vi "test_F9P_fgv-ver.vi"() -> ()   [LabVIEW 2019] (continued)
3,28,14,13,11,33,08,10,,,,,,1.19,0.67,0.98,4*09\r\n$GPGSV,4,1,13,02,65,334,42,04,08,037,40,05,48,261,36,06,58,076,45,1*6E\r\n$GPGSV,4,2,13,07,06,105,28,09,38,057,42,12,18,263,24,13,08,191,23,1*60\r\n$GPGSV,4,3,13,17,19,158,26,19,37,161,32,25,11,294,,29,07,323,19,1*62\r\n$GPGSV,4,4,13,30,01,134,,1*52\r\n$GPGSV,4,1,13,02,65,334,,04,08,037,30,05,48,261,32,06,58,076,34,6*6A\r\n$GPGSV,4,2,13,07,06,105,,09,38,057,35,12,18,263,12,13,08,191,,6*69\r\n$GPGSV,4,3,13,17,19,158,17,19,37,161,,25,11,294,,29,07,323,,6*6E\r\n$GPGSV,4,4,13,30,01,134,,6*55\r\n$GLGSV,2,1,06,70,55,030,35,71,68,223,28,72,17,216,42,84,09,133,10,1*7B\r\n$GLGSV,2,2,06,85,63,111,31,86,51,337,,1*78\r\n$GLGSV,2,1,06,70,55,030,,71,68,223,18,72,17,216,24,84,09,133,08,3*75\r\n$GLGSV,2,2,06,85,63,111,25,86,51,337,,3*7F\r\n$GAGSV,3,1,09,02,04,287,09,04,68,085,36,09,44,196,28,11,78,037,39,7*74\r\n$GAGSV,3,2,09,12,32,114,31,18,55,284,35,19,17,042,37,25,01,241,,7*73\r\n$GAGSV,3,3,09,36,35,314,23,7*4E\r\n$GAGSV,3,1,09,02,04,287,,04,68,085,35,09,44,196,26,11,78,037,33,2*7F\r\n$GAGSV,3,2,09,12,32,114,35,18,55,284,31,19,17,042,29,25,01,241,,2*79\r\n$GAGSV,3,3,09,36,35,314,26,2*4E\r\n$GBGSV,4,1,13,04,35,133,,05,09,257,,06,27,182,,07,09,201,21,1*78\r\n$GBGSV,4,2,13,08,65,355,40,09,07,194,,10,16,222,23,11,38,142,31,1*77\r\n$GBGSV,4,3,13,13,50,314,38,14,77,038,42,28,58,310,37,33,72,237,30,1*70\r\n$GBGSV,4,4,13,34,13,141,,1*45\r\n$GBGSV,4,1,13,04,35,133,,05,09,257,,06,27,182,,07,09,201,,3*79\r\n$GBGSV,4,2,13,08,65,355,39,09,07,194,,10,16,222,21,11,38,142,33,3*7B\r\n$GBGSV,4,3,13,13,50,314,39,14,77,038,36,28,58,310,,33,72,237,,3*77\r\n$GBGSV,4,4,13,34,13,141,,3*47\r\n$GNGLL,3723.61598,N,12656.96764,E,064242.00,A,A*7B\r\n$GNRMC,064243.00,A,3723.61604,N,12656.96767,E,0.173,,250720,,,A,V*1B\r\n$GNVTG,,T,,M,0.173,N,0.321,K,A*38\r\n$GNGGA,064243.00,3723.61604,N,12656.96767,E,1,12,0.65,41.5,M,18.5,M,,*76\r\n$GNGSA,A,3,17,19,06,05,02,12,09,,,,,,1.18,0.65,0.98,1*0E\r\n$GNGSA,A,3,85,70,71,72,,,,,,,,,1.18,0.65,0.98,2*01\r\n$GNGSA,A,3,36,19,11,04,09,12,,,,,,,1.18,0.65,0.98,3*0A\r\n$GNGSA,A,3,28,14,13,11,33,08,10,,,,,,1.18,0.65,0.98,4*0A\r\n$GPGSV,4,1,13,02,65,334,42,04,08,037,39,05,48,261,36,06,58,076,45,1*60\r\n$GPGSV,4,2,13,07,06,105,28,09,38,057,42,12,18,263,23,13,08,191,24,1*60\r\n$GPGSV,4,3,13,17,19,158,25,19,37,161,33,25,11,294,,29,07,323,17,1*6E\r\n$GPGSV,4,4,13,30,01,134,,1*52\r\n$GPGSV,4,1,13,02,65,334,,04,08,037,23,05,48,261,32,06,58,076,34,6*68\r\n$GPGSV,4,2,13,07,06,105,,09,38,057,34,12,18,263,11,13,08,191,,6*6B\r\n$GPGSV,4,3,13,17,19,158,22,19,37,161,,25,11,294,,29,07,323,,6*68\r\n$GPGSV,4,4,13,30,01,134,,6*55\r\n$GLGSV,2,1,06,70,55,030,34,71,68,223,27,72,17,216,42,84,09,133,15,1*70\r\n$GLGSV,2,2,06,85,63,111,29,86,51,337,,1*71\r\n$GLGSV,2,1,06,70,55,030,,71,68,223,14,72,17,216,24,84,09,133,11,3*71\r\n$GLGSV,2,2,06,85,63,111,26,86,51,337,,3*7C\r\n$GAGSV,3,1,09,02,04,287,06,04,68,085,36,09,44,196,25,11,78,037,39,7*76\r\n$GAGSV,3,2,09,12,32,114,35,18,55,284,37,19,17,042,34,25,01,241,,7*76\r\n$GAGSV,3,3,09,36,35,314,22,7*4F\r\n$GAGSV,3,1,09,02,04,287,,04,68,085,35,09,44,196,26,11,78,037,29,2*74\r\n$GAGSV,3,2,09,12,32,114,29,18,55,284,33,19,17,042,28,25,01,241,,2*77\r\n$GAGSV,3,3,09,36,35,314,27,2*4F\r\n$GBGSV,4,1,13,04,35,133,,05,09,257,,06,27,182,,07,09,201,19,1*73\r\n$GBGSV,4,2,13,08,65,355,40,09,07,194,,10,16,222,25,11,38,142,33,1*73\r\n$GBGSV,4,3,13,13,50,314,36,14,77,038,42,28,58,310,36,33,72,237,25,1*7B\r\n$GBGSV,4,4,13,34,13,141,,1*45\r\n$GBGSV,4,1,13,04,35,133,,05,09,257,,06,27,182,,07,09,201,,3*79\r\n$GBGSV,4,2,13,08,65,355,38,09,07,194,,10,16,222,21,11,38,142,33,3*7A\r\n$GBGSV,4,3,13,13,50,314,39,14,77,038,35,28,58,310,,33,72,237,,3*74\r\n$GBGSV,4,4,13,34,13,141,,3*47\r\n$GNGLL,3723.61604,N,12656.96767,E,064243.00,A,A*7F\r\n$GNRMC,064244.00,A,3723.61613,N,12656.96767,E,0.073,,250720,,,A,V*1B\r\n$GNVTG,,T,,M,0.073,N,0.135,K,A*3E\r\n$GNGGA,064244.00,3723.61613,N,12656.96767,E,1,12,0.63,41.5,M,18.5,M,,*71\r\n$GNGSA,A,3,17,19,06,05,02,12,09,,,,,,1.11,0.63,0.91,1*08\r\n$GNGSA,A,3,85,70,71,72,,,,,,,,,1.11,0.63,0.91,2*07\r\n$GNGSA,A,3,36,19,11,04,09,12,,,,,,,1.11,0.63,0.91,3*0C\r\n$GNGSA,A,3,28,14,13,11,33,08,10,,,,,,1.11,0.63,0.91,4*0C\r\n$GPGSV,4,1,13,02,65,334,43,04,08,037,39,05,48,261,38,06,58,076,45,1*6F\r\n$GPGSV,4,2,13,07,06,105,27,09,38,057,44,12,18,263,26,13,08,191,24,1*6C\r\n$GPGSV,4,3,13,17,19,158,24,19,37,161,33,25,11,294,,29,07,323,17,1*6F\r\n$GPGSV,4,4,13,30,01,134,,1*52\r\n$GPGSV,4,1,13,02,65,334,,04,08,037,24,05,48,261,33,06,58,076,33,6*69\r\n$GPGSV,4,2,13,07,06,105,,09,38,057,34,12,18,263,15,13,08,191,,6*6F\r\n$GPGSV,4,3,13,17,19,158,22,19,37,161,,25,11,294,,29,07,323,,6*68\r\n$GPGSV,4,4,13,30,01,134,,6*55\r\n$GLGSV,2,1,06,70,55,030,36,71,68,223,32,72,17,216,44,84,09,133,16,1*73\r\n$GLGSV,2,2,06,85,63,111,21,86,51,337,,1*79\r\n$GLGSV,2,1,06,70,55,030,,71,68,223,12,72,17,216,23,84,09,133,11,3*70\r\n$GLGSV,2,2,06,85,63,111,26,86,51,337,,3*7C\r\n$GAGSV,3,1,09,02,04,287,11,04,68,085,33,09,44,196,24,11,78,037,37,7*7A\r\n$GAGSV,3,2,09,12,32,114,32,18,55,284,39,19,17,042,35,25,01,241,,7*7E\r\n$GAGSV,3,3,09,36,35,314,20,7*4D\r\n$GAGSV,3,1,09,02,04,287,,04,68,085,34,09,44,196,25,11,78,037,31,2*7F\r\n$GAGSV,3,2,09,12,32,114,29,18,55,284,33,19,17,042,26,25,01,241,,2*79\r\n$GAGSV,3,3,09,36,35,314,29,2*41\r\n$GBGSV,4,1,13,04,35,133,,05,09,257,,06,27,182,,07,09,201,19,1*73\r\n$GBGSV,4,2,13,08,65,355,42,09,07,194,,10,16,222,25,11,37,142,32,1*7F\r\n$GBGSV,4,3,13,13,50,314,36,14,77,038,42,28,58,310,35,33,72,237,25,1*78\r\n$GBGSV,4,4,13,34,13,141,,1*45\r\n$GBGSV,4,1,13,04,35,133,,05,09,257,,06,27,182,,07,09,201,,3*79\r\n$GBGSV,4,2,13,08,65,355,37,09,07,194,,10,16,222,21,11,37,142,34,3*7D\r\n$GBGSV,4,3,13,13,50,314,39,14,77,038,35,28,58,310,,33,72,237,,3*74\r\n$GBGSV,4,4,13,34,13,141,,3*47\r\n$GNGLL,3723.61613,N,12656.96767,E,064244.00,A,A*7E\r\n$GNRMC,064245.00,A,3723.61615,N,12656.96774,E,0.035,,250720,,,A,V*1C\r\n$GNVTG,,T,,M,0.035,N,0.064,K,A*39\r\n$GNGGA,064245.00,3723.61615,N,12656.96774,E,1,12,0.65,41.6,M,18.5,M,,*71\r\n$GNGSA,A,3,17,19,06,05,02,12,09,,,,,,1.12,0.65,0.91,1*0D\r\n$GNGSA,A,3,85,70,71,72,,,,,,,,,1.12,0.65,0.91,2*02\r\n$GNGSA,A,3,36,19,11,04,09,12,,,,,,,1.12,0.65,0.91,3*09\r\n$GNGSA,A,3,28,14,13,11,33,08,10,,,,,,1.12,0.65,0.91,4*09\r\n$GPGSV,4,1,13,02,65,334,41,04,08,037,41,05,48,261,35,06,58,076,44,1*6E\r\n$GPGSV,4,2,13,07,06,105,25,09,38,057,42,12,18,263,26,13,08,191,25,1*69\r\n$GPGSV,4,3,13,17,19,158,26,19,37,161,33,25,11,294,,29,07,323,17,1*6D\r\n$GPGSV,4,4,13,30,01,134,,1*52\r\n$GPGSV,4,1,13,02,65,334,,04,08,037,26,05,48,261,33,06,58,076,33,6*6B\r\n$GPGSV,4,2,13,07,06,105,,09,38,057,33,12,18,263,17,13,08,191,,6*6A\r\n$GPGSV,4,3,13,17,19,158,22,19,37,161,,25,11,294,,29,07,323,,6*68\r\n$GPGSV,4,4,13,30,01,134,,6*55\r\n$GLGSV,2,1,06,70,55,030,35,71,68,223,26,72,17,216,44,84,09,133,08,1*7A\r\n$GLGSV,2,2,06,85,63,111,31,86,51,337,,1*78\r\n$GLGSV,2,1,06,70,55,030,,71,68,223,08,72,17,216,23,84,09,133,09,3*72\r\n$GLGSV,2,2,06,85,63,111,27,86,51,337,,3*7D\r\n$GAGSV,3,1,09,02,04,287,08,04,68,085,37,09,44,196,21,11,78,037,38,7*7C\r\n$GAGSV,3,2,09,12,32,114,35,18,55,284,38,19,17,042,35,25,01,241,,7*78\r\n$GAGSV,3,3,09,36,35,314,21,7*4C\r\n$GAGSV,3,1,09,02,04,287,,04,68,085,34,09,44,196,25,11,78,037,31,2*7F\r\n$GAGSV,3,2,09,12,32,114,30,18,55,284,33,19,17,042,25,25,01,241,,2*72\r\n$GAGSV,3,3,09,36,35,314,29,2*41\r\n$GBGSV,4,1,13,04,35,133,,05,09,257,,06,27,182,,07,09,201,19,1*73\r\n$GBGSV,4,2,13,08,65,355,41,09,07,194,,10,16,222,26,11,37,142,33,1*7E\r\n$GBGSV,4,3,13,13,50,315,36,14,77,038,42,28,58,310,35,33,72,237,32,1*7F\r\n$GBGSV,4,4,13,34,13,141,,1*45\r\n$GBGSV,4,1,13,04,35,133,,05,09,257,,06,27,182,,07,09,201,,3*79\r\n$GBGSV,4,2,13,08,65,355,38,09,07,194,,10,16,222,21,11,37,142,34,3*72\r\n$GBGSV,4,3,13,13,50,315,39,14,77,038,35,28,58,310,,33,72,237,,3*75\r\n$GBGSV,4,4,13,34,13,141,,3*47\r\n$GNGLL,3723.61615,N,12656.96774,E,064245.00,A,A*7B\r\n$GNRMC,064246.00,A,3723.61615,N,12656.96777,E,0.050,,250720,,,A,V*1F\r\n$GNVTG,,T,,M,0.050,N,0.092,K,A*33\r\n$GNGGA,064246.00,3723.61615,N,12656.96777,E,1,12,0.63,41.6,M,18.5,M,,*77\r\n$GNGSA,A,3,17,19,06,05,02,12,09,,,,,,1.11,0.63,0.91,1*08\r\n$GNGSA,A,3,85,70,71,72,,,,,,,,,1.11,0.63,0.91,2*07\r\n$GNGSA,A,3,36,19,11,04,09,12,,,,,,,1.11,0.63,0.91,3*0C\r\n$GNGSA,A,3,28,14,13,11,33,08,10,,,,,,1.11,0.63,0.91,4*0C\r\n$GPGSV,4,1,13,02,65,334,40,04,08,037,39,05,48,261,37,06,58,076,45,1*63\r\n$GPGSV,4,2,13,07,06,105,,09,38,057,43,12,18,263,26,13,08,191,26,1*6C\r\n$GPGSV,4,3,13,17,19,158,26,19,37,161,34,25,11,294,,29,07,323,15,1*68\r\n$GPGSV,4,4,13,30,01,134,,1*52\r\n$GPGSV,4,1,13,02,65,334,,04,08,037,26,05,48,261,33,06,58,076,34,6*6C\r\n$GPGSV,4,2,13,07,06,105,,09,38,057,35,12,18,263,16,13,08,191,,6*6D\r\n$GPGSV,4,3,13,17,19,158,23,19,37,161,,25,11,294,,29,07,323,,6*69\r\n$GPGSV,4,4,13,30,01,134,,6*55\r\n$GLGSV,2,1,06,70,55,030,36,71,68,223,22,72,17,216,44,84,09,133,09,1*7C\r\n$GLGSV,2,2,06,85,63,111,31,86,51,337,,1*78\r\n$GLGSV,2,1,06,70,55,030,,71,68,223,19,72,17,216,23,84,09,133,08,3*73\r\n$GLGSV,2,2,06,85,63,111,27,86,51,337,,3*7D\r\n$GAGSV,3,1,09,02,04,287,11,04,68,085,36,09,44,196,24,11,78,037,38,7*70\r\n$GAGSV,3,2,09,12,32,114,36,18,55,284,39,19,17,042,34,25,01,241,,7*7B\r\n$GAGSV,3,3,09,36,35,314,22,7*4F\r\n$GAGSV,3,1,09,02,04,287,,04,68,085,34,09,44,196,25,11,78,037,31,2*7F\r\n$GAGSV,3,2,09,12,32,114,29,18,55,284,34,19,17,042,26,25,01,241,,2*7E\r\n$GAGSV,3,3,09,36,35,314,29,2*41\r\n$GBGSV,4,1,13,04,35,133,,05,09,257,,06,27,182,,07,09,201,19,1*73\r\n$GBGSV,4,2,13,08,65,355,41,09,07,194,,10,16,222,26,11,37,142,32,1*7F\r\n$GBGSV,4,3,13,13,50,315,36,14,76,037,41,28,58,310,36,33,72,237,29,1*7B\r\n$GBGSV,4,4,13,34,13,141,,1*45\r\n$GBGSV,4,1,13,04,35,133,,05,09,257,,06,27,182,,07,09,201,,3*79\r\n$GBGSV,4,2,13,08,65,355,38,09,07,194,,10,16,222,21,11,37,142,34,3*72\r\n$GBGSV,4,3,13,13,50,315,39,14,76,037,36,28,58,310,,33,72,237,,3*78\r\n$GBGSV,4,4,13,34,13,141,,3*47\r\n$GNGLL,3723.61615,N,12656.96777,E,064246.00,A,A*7B\r\n$GNRMC,064247.00,A,3723.61615,N,12656.96784,E,0.008,,250720,,,A,V*1F\r\n$GNVTG,,T,,M,0.008,N,0.015,K,A*31\r\n$GNGGA,064247.00,3723.61615,N,12656.96784,E,1,12,0.63,41.8,M,18.5,M,,*74\r\n$GNGSA,A,3,17,19,06,05,02,12,09,,,,,,1.11,0.63,0.91,1*08\r\n$GNGSA,A,3,85,70,71,72,,,,,,,,,1.11,0.63,0.91,2*07\r\n$GNGSA,A,3,36,19,11,04,09,12,,,,,,,1.11,0.63,0.91,3*0C\r\n$GNGSA,A,3,28,14,13,11,33,08,10,,,,,,1.11,0.63,0.91,4*0C\r\n$GPGSV,4,1,13,02,65,334,41,04,08,037,40,05,48,261,36,06,58,076,44,1*6C\r\n$GPGSV,4,2,13,07,06,105,,09,38,057,43,12,18,263,27,13,08,191,26,1*6D\r\n$GPGSV,4,3,13,17,19,158,,19,37,161,34,25,11,294,,29,07,323,13,1*6A\r\n$GPGSV,4,4,13,30,01,134,,1*52\r\n$GPGSV,4,1,13,02,65,334,,04,08,037,24,05,48,261,32,06,58,076,34,6*6F\r\n$GPGSV,4,2,13,07,06,105,,09,38,057,35,12,18,263,16,13,08,191,,6*6D\r\n$GPGSV,4,3,13,17,19,158,25,19,37,161,,25,11,294,,29,07,323,,6*6F\r\n$GPGSV,4,4,13,30,01,134,,6*55\r\n$GLGSV,2,1,06,70,55,030,36,71,68,223,21,72,17,216,43,84,09,133,09,1*78\r\n$GLGSV,2,2,06,85,63,111,31,86,51,337,,1*78\r\n$GLGSV,2,1,06,70,55,030,,71,68,223,18,72,17,216,26,84,09,133,10,3*7E\r\n$GLGSV,2,2,06,85,63,111,29,86,51,337,,3*73\r\n$GAGSV,3,1,09,02,04,287,07,04,68,085,37,09,44,196,25,11,78,037,38,7*77\r\n$GAGSV,3,2,09,12,32,114,37,18,55,284,38,19,17,042,33,25,01,241,,7*7C\r\n$GAGSV,3,3,09,36,35,314,23,7*4E\r\n$GAGSV,3,1,09,02,04,287,,04,68,085,33,09,44,196,25,11,78,037,30,2*79\r\n$GAGSV,3,2,09,12,32,114,28,18,55,284,34,19,17,042,25,25,01,241,,2*7C\r\n$GAGSV,3,3,09,36,35,314,29,2*41\r\n$GBGSV,4,1,13,04,35,133,,05,09,257,,06,27,182,,07,09,201,18,1*72\r\n$GBGSV,4,2,13,08,65,355,41,09,07,194,,10,16,222,25,11,37,142,33,1*7D\r\n$GBGSV,4,3,13,13,50,315,35,14,76,037,42,28,58,310,36,33,72,237,29,1*7B\r\n$GBGSV,4,4,13,34,13,141,,1*45\r\n$GBGSV,4,1,13,04,35,133,,05,09,257,,06,27,182,,07,09,201,,3*79\r\n$GBGSV,4,2,13,08,65,355,37,09,07,194,,10,16,222,21,11,37,142,34,3*7D\r\n$GBGSV,4,3,13,13,50,315,39,14,76,037,35,28,58,310,,33,72,237,,3*7B\r\n$GBGSV,4,4,13,34,13,141,,3*47\r\n$GNGLL,3723.61615,N,12656.96784,E,064247.00,A,A*76\r\n$GNRMC,064248.00,A,3723.61617,N,12656.96789,E,0.013,,250720,,,A,V*15\r\n$GNVTG,,T,,M,0.013,N,0.024,K,A*39\r\n$GNGGA,064248.00,3723.61617,N,12656.96789,E,1,12,0.63,41.9,M,18.5,M,,*75\r\n$GNGSA,A,3,17,19,06,05,02,12,09,,,,,,1.11,0.63,0.91,1*08\r\n$GNGSA,A,3,85,70,71,72,,,,,,,,,1.11,0.63,0.91,2*07\r\n$GNGSA,A,3,36,19,11,04,09,12,,,,,,,1.11,0.63,0.91,3*0C\r\n$GNGSA,A,3,28,14,13,11,33,08,10,,,,,,1.11,0.63,0.91,4*0C\r\n$GPGSV,4,1,13,02,65,334,43,04,08,037,38,05,48,261,38,06,58,076,45,1*6E\r\n$GPGSV,4,2,13,07,06,105,,09,38,057,44,12,18,263,29,13,08,191,26,1*64\r\n$GPGSV,4,3,13,17,19,158,27,19,37,161,34,25,11,294,,29,07,323,12,1*6E\r\n$GPGSV,4,4,13,30,01,134,,1*52\r\n$GPGSV,4,1,13,02,65,334,,04,08,037,22,05,48,261,32,06,58,076,35,6*68\r\n$GPGSV,4,2,13,07,06,105,,09,38,057,35,12,18,263,16,13,08,191,,6*6D\r\n$GPGSV,4,3,13,17,19,158,26,19,37,161,,25,11,294,,29,07,323,,6*6C\r\n$GPGSV,4,4,13,30,01,134,,6*55\r\n$GLGSV,2,1,06,70,55,030,37,71,68,223,21,72,17,216,44,84,09,133,09,1*7E\r\n$GLGSV,2,2,06,85,63,111,32,86,51,337,,1*7B\r\n$GLGSV,2,1,06,70,55,030,,71,68,223,18,72,17,216,26,84,09,133,09,3*76\r\n$GLGSV,2,2,06,85,63,111,30,86,51,337,,3*7B\r\n$GAGSV,3,1,09,02,04,287,08,04,68,085,36,09,44,196,25,11,78,037,38,7*79\r\n$GAGSV,3,2,09,12,32,114,36,18,55,284,39,19,17,042,32,25,01,241,,7*7D\r\n$GAGSV,3,3,09,36,35,314,23,7*4E\r\n$GAGSV,3,1,09,02,04,287,,04,68,085,33,09,44,196,25,11,78,037,30,2*79\r\n$GAGSV,3,2,09,12,32,114,27,18,55,284,34,19,17,042,26,25,01,241,,2*70\r\n$GAGSV,3,3,09,36,35,314,29,2*41\r\n$GBGSV,4,1,13,04,35,133,,05,09,257,,06,27,182,,07,09,201,19,1*73\r\n$GBGSV,4,2,13,08,65,355,41,09,07,194,,10,16,222,25,11,37,142,33,1*7D\r\n$GBGSV,4,3,13,13,50,315,35,14,76,037,41,28,58,310,36,33,72,237,29,1*78\r\n$GBGSV,4,4,13,34,13,141,,1*45\r\n$GBGSV,4,1,13,04,35,133,,05,09,257,,06,27,182,,07,09,201,,3*79\r\n$GBGSV,4,2,13,08,65,355,37,09,07,194,,10,16,222,21,11,37,142,33,3*7A\r\n$GBGSV,4,3,13,13,50,315,39,14,76,037,35,28,58,310,,33,72,237,,3*7B\r\n$GBGSV,4,4,13,34,13,141,,3*47\r\n$GNGLL,3723.61617,N,12656.96789,E,064248.00,A,A*76\r\n$GNRMC,064249.00,A,3723.61623,N,12656.96795,E,0.056,,250720,,,A,V*1F\r\n$GNVTG,,T,,M,0.056,N,0.103,K,A*3C\r\n$GNGGA,064249.00,3723.61623,N,12656.96795,E,1,12,0.62,42.2,M,18.5,M,,*77\r\n$GNGSA,A,3,17,19,06,05,02,12,09,,,,,,1.07,0.62,0.88,1*06\r\n$GNGSA,A,3,85,70,71,72,,,,,,,,,1.07,0.62,0.88,2*09\r\n$GNGSA,A,3,36,19,11,04,09,12,,,,,,,1.07,0.62,0.88,3*02\r\n$GNGSA,A,3,28,14,13,11,33,08,10,,,,,,1.07,0.62,0.88,4*02\r\n$GPGSV,4,1,13,02,65,334,42,04,08,037,39,05,48,261,38,06,58,076,44,1*6F\r\n$GPGSV,4,2,13,07,06,105,,09,38,057,44,12,18,263,30,13,08,191,25,1*6F\r\n$GPGSV,4,3,13,17,19,158,25,19,37,161,34,25,11,294,,29,07,323,13,1*6D\r\n$GPGSV,4,4,13,30,01,134,,1*52\r\n$GPGSV,4,1,13,02,65,334,,04,08,037,23,05,48,261,32,06,58,076,36,6*6A\r\n$GPGSV,4,2,13,07,06,105,,09,38,057,35,12,18,263,16,13,08,191,,6*6D\r\n$GPGSV,4,3,13,17,19,158,26,19,37,161,,25,11,294,,29,07,323,,6*6C\r\n$GPGSV,4,4,13,30,01,134,,6*55\r\n$GLGSV,2,1,06,70,55,030,37,71,68,223,20,72,17,216,44,84,09,133,10,1*77\r\n$GLGSV,2,2,06,85,63,111,32,86,51,337,,1*7B\r\n$GLGSV,2,1,06,70,55,030,,71,68,223,19,72,17,216,26,84,09,133,11,3*7E\r\n$GLGSV,2,2,06,85,63,111,30,86,51,337,,3*7B\r\n$GAGSV,3,1,09,02,04,287,09,04,68,085,37,09,44,196,24,11,78,037,38,7*78\r\n$GAGSV,3,2,09,12,32,114,36,18,55,284,39,19,17,042,32,25,01,241,,7*7D\r\n$GAGSV,3,3,09,36,35,314,25,7*48\r\n$GAGSV,3,1,09,02,04,287,,04,68,085,33,09,44,196,25,11,78,037,30,2*79\r\n$GAGSV,3,2,09,12,32,114,26,18,55,284,34,19,17,042,26,25,01,241,,2*71\r\n$GAGSV,3,3,09,36,35,314,29,2*41\r\n$GBGSV,4,1,13,04,35,133,,05,09,257,,06,27,182,,07,09,201,20,1*79\r\n$GBGSV,4,2,13,08,65,355,41,09,07,194,,10,16,222,26,11,37,142,32,1*7F\r\n$GBGSV,4,3,13,13,50,315,35,14,76,037,41,28,58,310,36,33,72,237,28,1*79\r\n$GBGSV,4,4,13,34,13,141,,1*45\r\n$GBGSV,4,1,13,04,35,133,,05,09,257,,06,27,182,,07,09,201,,3*79\r\n$GBGSV,4,2,13,08,65,355,37,09,07,194,,10,16,222,20,11,37,142,33,3*7B\r\n$GBGSV,4,3,13,13,50,315,39,14,76,037,34,28,58,310,,33,72,237,,3*7A\r\n$GBGSV,4,4,13,34,13,141,,3*47\r\n$GNGLL,3723.61623,N,12656.96795,E,064249.00,A,A*7D\r\n$GNRMC,064250.00,A,3723.61635,N,12656.96804,E,0.009,,250720,,,A,V*1D\r\n$GNVTG,,T,,M,0.009,N,0.016,K,A*33\r\n$GNGGA,064250.00,3723.61635,N,12656.96804,E,1,12,0.61,42.5,M,18.5,M,,*7B\r\n$GNGSA,A,3,17,19,06,05,02,12,09,,,,,,1.08,0.61,0.89,1*0B\r\n$GNGSA,A,3,85,70,71,72,,,,,,,,,1.08,0.61,0.89,2*04\r\n$GNGSA,A,3,36,19,11,04,09,12,,,,,,,1.08,0.61,0.89,3*0F\r\n$GNGSA,A,3,28,14,13,11,33,08,10,,,,,,1.08,0.61,0.89,4*0F\r\n$GPGSV,4,1,13,02,65,334,42,04,08,037,41,05,48,261,36,06,58,076,45,1*6F\r\n$GPGSV,4,2,13,07,06,105,,09,38,057,44,12,18,263,31,13,08,191,25,1*6E\r\n$GPGSV,4,3,13,17,19,158,,19,37,161,34,25,11,294,26,29,07,323,15,1*68\r\n$GPGSV,4,4,13,30,01,134,,1*52\r\n$GPGSV,4,1,13,02,65,334,,04,08,037,23,05,48,261,32,06,58,076,36,6*6A\r\n$GPGSV,4,2,13,07,06,105,,09,38,057,36,12,18,263,16,13,08,191,,6*6E\r\n$GPGSV,4,3,13,17,19,158,26,19,37,161,,25,11,294,,29,07,323,,6*6C\r\n$GPGSV,4,4,13,30,01,134,,6*55\r\n$GLGSV,2,1,06,70,55,030,37,71,68,223,22,72,17,216,44,84,09,133,12,1*77\r\n$GLGSV,2,2,06,85,63,111,32,86,51,337,,1*7B\r\n$GLGSV,2,1,06,70,55,030,,71,68,223,19,72,17,216,26,84,09,133,10,3*7F\r\n$GLGSV,2,2,06,85,63,111,30,86,51,337,,3*7B\r\n$GAGSV,3,1,09,02,04,287,08,04,68,085,37,09,44,196,24,11,78,037,38,7*79\r\n$GAGSV,3,2,09,12,32,115,36,18,55,284,39,19,17,042,31,25,01,241,,7*7F\r\n$GAGSV,3,3,09,36,35,314,26,7*4B\r\n$GAGSV,3,1,09,02,04,287,,04,68,085,33,09,44,196,24,11,78,037,30,2*78\r\n$GAGSV,3,2,09,12,32,115,26,18,55,284,34,19,17,042,26,25,01,241,,2*70\r\n$GAGSV,3,3,09,36,35,314,28,2*40\r\n$GBGSV,4,1,13,04,35,133,,05,09,257,,06,27,182,,07,09,201,20,1*79\r\n$GBGSV,4,2,13,08,65,355,41,09,07,194,,10,16,222,27,11,37,142,32,1*7E\r\n$GBGSV,4,3,13,13,50,315,34,14,76,037,41,28,59,310,36,33,72,237,29,1*78\r\n$GBGSV,4,4,13,34,13,141,,1*45\r\n$GBGSV,4,1,13,04,35,133,,05,09,257,,06,27,182,,07,09,201,,3*79\r\n$GBGSV,4,2,13,08,65,355,37,09,07,194,,10,16,222,20,11,37,142,33,3*7B\r\n$GBGSV,4,3,13,13,50,315,39,14,76,037,34,28,59,310,,33,72,237,,3*7B\r\n$GBGSV,4,4,13,34,13,141,,3*47\r\n$GNGLL,3723.61635,N,12656.96804,E,064250.00,A,A*75\r\n$GNRMC,064251.00,A,3723.61643,N,12656.96813,E,0.042,,250720,,,A,V*14\r\n$GNVTG,,T,,M,0.042,N,0.078,K,A*34\r\n$GNGGA,064251.00,3723.61643,N,12656.96813,E,1,12,0.63,42.9,M,18.5,M,,*73\r\n$GNGSA,A,3,17,19,06,05,02,12,09,,,,,,1.09,0.63,0.89,1*08\r\n$GNGSA,A,3,85,70,71,72,,,,,,,,,1.09,0.63,0.89,2*07\r\n$GNGSA,A,3,36,19,11,04,09,12,,,,,,,1.09,0.63,0.89,3*0C\r\n$GNGSA,A,3,28,14,13,11,33,08,10,,,,,,1.09,0.63,0.89,4*0C\r\n$GPGSV,4,1,13,02,65,334,44,04,08,037,41,05,48,261,36,06,58,076,44,1*68\r\n$GPGSV,4,2,13,07,06,105,,09,38,057,45,12,18,263,31,13,08,191,24,1*6E\r\n$GPGSV,4,3,13,17,19,158,22,19,37,161,34,25,11,294,25,29,07,323,17,1*69\r\n$GPGSV,4,4,13,30,01,134,,1*52\r\n$GPGSV,4,1,13,02,65,334,,04,08,037,26,05,48,261,32,06,58,076,36,6*6F\r\n$GPGSV,4,2,13,07,06,105,,09,38,057,36,12,18,263,17,13,08,191,,6*6F\r\n$GPGSV,4,3,13,17,19,158,25,19,37,161,,25,11,294,,29,07,323,,6*6F\r\n$GPGSV,4,4,13,30,01,134,,6*55\r\n$GLGSV,2,1,06,70,55,030,37,71,68,223,25,72,17,216,43,84,09,133,11,1*74\r\n$GLGSV,2,2,06,85,63,111,26,86,51,337,,1*7E\r\n$GLGSV,2,1,06,70,55,030,,71,68,223,19,72,17,216,26,84,09,133,08,3*76\r\n$GLGSV,2,2,06,85,63,111,29,86,51,337,,3*73\r\n$GAGSV,3,1,09,02,04,287,06,04,68,085,37,09,44,196,23,11,78,037,39,7*71\r\n$GAGSV,3,2,09,12,32,115,35,18,55,284,40,19,17,042,31,25,01,241,,7*72\r\n$GAGSV,3,3,09,36,35,314,26,7*4B\r\n$GAGSV,3,1,09,02,04,287,,04,68,085,33,09,44,196,23,11,78,037,30,2*7F\r\n$GAGSV,3,2,09,12,32,115,26,18,55,284,35,19,17,042,26,25,01,241,,2*71\r\n$GAGSV,3,3,09,36,35,314,28,2*40\r\n$GBGSV,4,1,13,04,35,133,,05,09,257,,06,27,182,,07,09,201,19,1*73\r\n$GBGSV,4,2,13,08,65,355,41,09,07,194,,10,16,222,27,11,37,142,33,1*7F\r\n$GBGSV,4,3,13,13,50,315,34,14,76,037,41,28,59,310,36,33,72,237,29,1*78\r\n$GBGSV,4,4,13,34,13,141,,1*45\r\n$GBGSV,4,1,13,04,35,133,,05,09,257,,06,27,182,,07,09,201,,3*79\r\n$GBGSV,4,2,13,08,65,355,37,09,07,194,,10,16,222,19,11,37,142,33,3*71\r\n$GBGSV,
